vi "NIMS_DF_fir_linf(m, f, mag, ripple).vi"(8 "ripple":dbl[](array[numeric]), 9 "mag":dbl[](array[numeric]), 10 "f":dbl[](array[numeric]), 11 "flag":enum32{"mineven", "minodd"}(ring)) -> (0 "error":i32, 3 "b":dbl[](array[numeric]))   [LabVIEW 2017, in "NI_DigFilter_MathScript.lvlib"]
uses:
  <vilib>/addons/Digital Filter Design/NI_DigFilter_MathScript.lvlib
  <vilib>/addons/Digital Filter Design/NI_DigFilterLicensed.lvlib
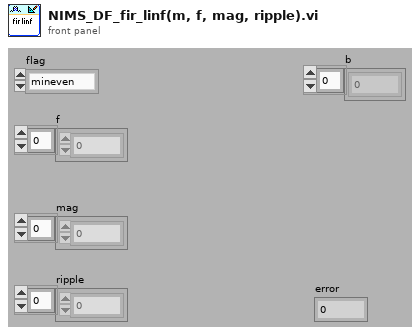
[diagram p1: front panel]
types:
  T1 = typedef "NI_DigFilterLicensed.lvlib/DFD Adv Band Spec.ctl" = cluster{"band specification":cluster{"freq":dbl, "amplitude":dbl, "weight":dbl}[], "ripple constraint":dbl}
  T2 = typedef "NI_DigFilterLicensed.lvlib/DFD Filter Obj.ctl" = cluster{"mSRate_Fs":dbl, "mSRate_Version":string, "mSRate_Comments":string, "mSRate_OrgCoef":T3, "mSRate_CurCoef":T3, "mSRate_Quantized?":bool, "mSRate_QCoef":T3, "mSRate_QSettings":T5[], "mSRate_Order":i32, "mSRate_Scaling":cluster{"mSRate_ScaleByPowerOf2?":bool, "mSRate_ScaleType":T7}}
  T3 = typedef "NI_DigFilterLicensed.lvlib/DFD Filter Coef.ctl" = cluster{"type":T4, "gain":dbl, "coef a (k)":dbl[], "coef b (v)":dbl[]}
  T4 = typedef "NI_DigFilterLicensed.lvlib/DFD Filter Structure Type Selector.ctl" = enum16{"Undefined", "FIR Direct Form", "FIR Direct Form Transposed", "FIR Symmetric", "FIR Antisymmetric", "IIR Direct Form I", "IIR Direct Form I Transposed", "IIR Direct Form II", "IIR Direct Form II Transposed", "IIR Cascaded Second Order Sections Form I", "IIR Cascaded Second Order Sections Form I Transposed", "IIR Cascaded Second Order Sections Form II", "IIR Cascaded Second Order Sections Form II Transposed", "Lattice Allpass (basic sections)", "Lattice Allpass (one multiplier sections)", "Lattice Allpass (normalized sections)", "Lattice AR (basic sections)", "Lattice AR (one multiplier sections)", "Lattice AR (normalized sections)", "Lattice MA (minimum phase)", "Lattice MA (maximum phase)", "Lattice ARMA (basic sections)", "Lattice ARMA (one multiplier sections)", "Lattice ARMA (normalized sections)"}
  T5 = typedef "NI_DigFilterLicensed.lvlib/dfd_Internal Quantization Settings.ctl" = cluster{"source":T6, "wl":i16, "iwl":i16, "overflow mode":enum16{"Saturation", "Wrap"}, "rounding mode":enum16{"Nearest", "Truncation"}, "signed?":bool}
  T6 = typedef "NI_DigFilterLicensed.lvlib/dfd_Internal Quantization Srcs.ctl" = u16
  T7 = typedef "NI_DigFilterLicensed.lvlib/DFD Coef Norm Type.ctl" = enum16{"No Norm", "Time Domain 1-Norm", "Time Domain 2-Norm", "Time Domain Inf-Norm"}
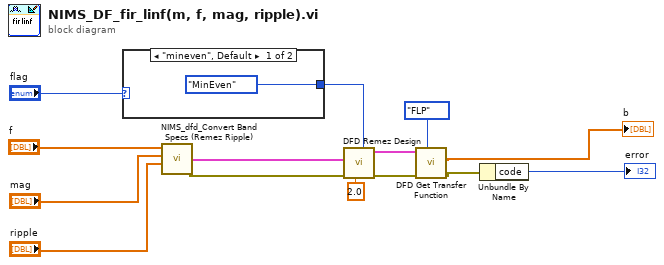
[diagram p0: block diagram]
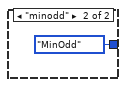
[diagram p2: hidden frame]
diagram:
  n1 = case shown="\"mineven\", Default" "flag" {
    tunnel: [enum32{"User Defined", "MinEven", "MinOdd"}."MinEven" ("minimum order") enum32{"User Defined", "MinEven", "MinOdd"}."MinOdd" ("minimum order")] -> w4
    frame "mineven", Default {
    }
    frame "minodd" {
    }
  }
  n2 = call <vilib>:"NIMS_dfd_Convert Band Specs (Remez Ripple).vi"("Ripple"="ripple", "A"="mag", "F"="f") -> ("error out"=w12:errorcluster, "band specs"=w13:T1[])  [unwired: 7 out]
  n3 = call <vilib>:"DFD Remez Design.vi"("minimum order"=w4, "fs [Hz]"=2.0, "error in (no error)"=w12, "band specs"=w13) -> ("error out"=w9:errorcluster, "filter out"=w10:T2)  [unwired: 3 in, 3 out]
  n4 = call <vilib>:"DFD Get Transfer Function.vi"("type (FLP)"=enum16{"FLP", "FXP"}."FLP", "error in (no error)"=w9, "filter in"=w10) -> ("error out"=w2:errorcluster, "numerator"=→"b":dbl[])  [unwired: 7 out]
  n5 = Unbundle By Name(w2) -> ("code"=→"error":i32)
